vi "addStartup.vi"(0 "object in":refnum<class "interface.lvclass">, 1 "启动文件路径":path, 5 "error in (no error)":errorcluster) -> (14 "object out":refnum<class "interface.lvclass">, 15 "添加成功标记":bool, 19 "error out":errorcluster)   [LabVIEW 2016, in "interface.lvclass"]
uses:
  interface.lvclass
  <vilib>/registry/registry.llb/Registry RtKey.ctl
  <vilib>/registry/registry.llb/Write Registry Value Simple STR.vi
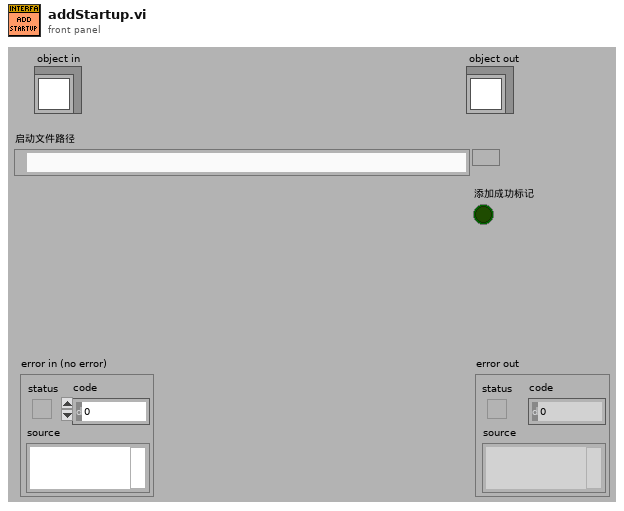
[diagram p1: front panel]
types:
  T1 = typedef "Registry RtKey.ctl" = enum32{"HKEY_CLASSES_ROOT", "HKEY_CURRENT_USER", "HKEY_LOCAL_MACHINE", "HKEY_USERS", "HKEY_PERFORMANCE_DATA", "HKEY_CURRENT_CONFIG", "HKEY_DYN_DATA"}
  T2 = typedef "Registry refnum.ctl" = refnum<k1>
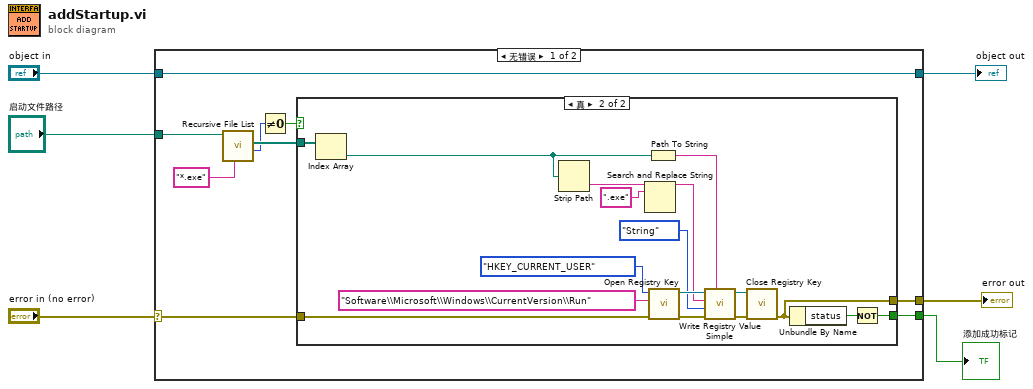
[diagram p0: block diagram]
diagram:
  n1 = case shown="无错误" "error in (no error)" {
    selector: "error in (no error)" -> [w9 w35]
    tunnel: [w8 w35] -> w5
    tunnel: [w7 w34] -> w3
    tunnel: "object in" -> [w7 w34]
    tunnel: "启动文件路径" -> [w11 _]
    tunnel: [w10 _] -> w1
    frame No Error {
      n2 = call <vilib>:"Recursive File List.vi"("pattern"="*.exe", "Folder Path"=w11) -> ("Number of Files"=w13:i32, "All Files in Dir"=w14:path[])  [unwired: 5 in, 3 out]
      n3 = Not Equal To 0?(x=w13) -> (x != 0?=w12:bool)
      n4 = case shown="真" w12 {
        tunnel: w14 -> [_ w33]
        tunnel: [_ w21] -> w10
        tunnel: w9 -> [w16 w18]
        tunnel: [w16 w17] -> w8
        frame False {
        }
        frame True {
          n5 = Index Array(array=w33) -> (element=w32:path)  [unwired: 1 in]
          n6 = Strip Path(path=w32) -> (name=w31:string)  [unwired: 1 out]
          n7 = Search and Replace String(input string=w31, search string=".exe" ("搜索字符串")) -> (result string=w19:string)  [unwired: 6 in, 3 out]
          n8 = Path To String(path=w32) -> (string=w20:string)
          n9 = call <vilib>:"Open Registry Key.vi"("error in (no error)"=w18, "subkey"="Software\\Microsoft\\Windows\\CurrentVersion\\Run", "root key (HKEY_LOCAL_MACHINE)"=Registry_RtKey."HKEY_CURRENT_USER") -> ("error out"=w27:errorcluster, "refnum out"=w26:T2)  [unwired: 7 in]
          n10 = call-poly <vilib>:"Write Registry Value Simple.vi"("String/Binary data"=w20, "error in (no error)"=w27, "simple data type"=enum16{"String", "Binary", "DWORD"}."String", "value"=w19, "refnum"=w26) -> ("error out"=w29:errorcluster, "refnum out"=w28:T2)  [unwired: 3 in]
          n11 = call <vilib>:"Close Registry Key.vi"("error in (no error)"=w29, "refnum"=w28) -> ("error out"=w17:errorcluster)  [unwired: 5 in]
          n12 = Unbundle By Name(w17) -> ("status"=w22:bool)
          n13 = Not(x=w22) -> (.not. x?=w21:bool)
        }
      }
    }
    frame Error {
    }
  }
  "error out" <- w5
  "object out" <- w3
  "添加成功标记" <- w1
